vi "test_2_调用子vi.vi"   [LabVIEW 2012]
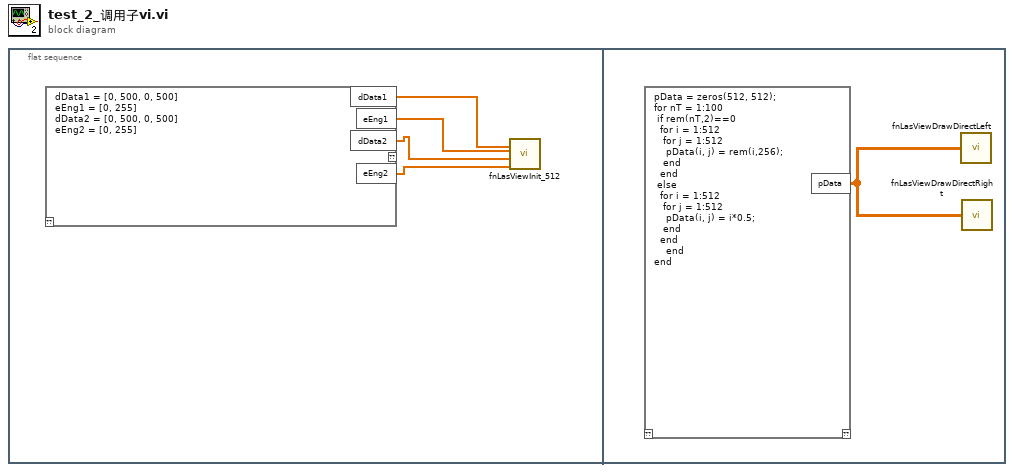
[diagram p0: block diagram]
diagram:
  n1 = flat-sequence {
    frame #0 {
      n2 = script code="dData1 = [0, 500, 0, 500]\neEng1 = [0, 255]\ndData2 = [0, 500, 0, 500]\neEng2 = [0, 255]"() -> ("dData1"=w4:cdb[], "eEng1"=w3:cdb[], "dData2"=w2:cdb[], "eEng2"=w1:cdb[])  [unwired: 1 in, 1 out]
      n3 = call "fnLasViewInit_512.vi"("eEng2"=w1, "dData2"=w2, "eEng1"=w3, "dData1"=w4) -> ()  [unwired: 1 out]
    }
    frame #1 {
      n4 = script code="pData = zeros(512, 512);\nfor nT = 1:100\n\tif rem(nT,2)==0\n\t\tfor i = 1:512\n\t\t\tfor j = 1:512\n\t\t\t\tpData(i, j) = rem(i,256);\n\t\t\tend\n\t\tend\n\telse\n\t\tfor i = 1:512\n\t\t\tfor j = 1:512\n\t\t\t\tpData(i, j) = i*0.5;\n\t\t\tend\n\t\tend\n    end\nend"() -> ("pData"=w5:cdb[][])  [unwired: 1 in, 1 out]
      n5 = call "fnLasViewDrawDirectLeft.vi"("pData"=w5) -> ()  [unwired: 1 out]
      n6 = call "fnLasViewDrawDirectRight.vi"("pData"=w5) -> ()  [unwired: 1 out]
    }
  }
